vi "Configure Function FFT.vi"(6 "FFT Window (Hanning)":string(combo)="HANN", 8 "error in (no error)":errorcluster {"code" format="%.0x"}, 9 "fft center (500.0E+3 Hz)":dbl=500000.0 caption="FFT Center (500.0E+3 Hz)" format="%^.2e", 10 "fft span (1.0E+6 hz)":dbl=1000000.0 caption="FFT Span (1.0E+6 Hz)" format="%^.2e", 11 "VISA Resource Name":refnum<visa-resource-name>) -> (0 "error out":errorcluster {"code" format="%.0x"}, 3 "VISA Resource Name Out":refnum<visa-resource-name>)   [LabVIEW 2011, in "Agilent 546XX Series.lvlib"]
doc: "This VI configures the span, center and window values for the FFT function.\n\nNote: This VI has effects on the instrument only if the function operation is set to FFT."
uses:
  Agilent 546XX Series.lvlib
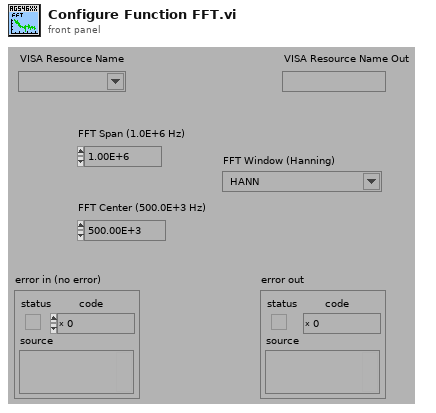
[diagram p1: front panel]
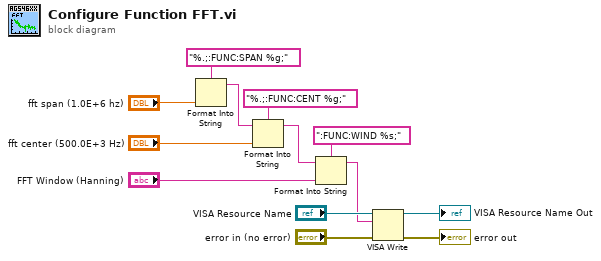
[diagram p0: block diagram]
diagram:
  n1 = Format Into String(format string="%.;:FUNC:SPAN %g;", "fft span (1.0E+6 hz)") -> (resulting string=w6:string)  [unwired: 2 in, 1 out]
  n2 = Format Into String(format string="%.;:FUNC:CENT %g;", initial string=w6, "fft center (500.0E+3 Hz)") -> (resulting string=w3:string)  [unwired: 1 in, 1 out]
  n3 = Format Into String(format string=":FUNC:WIND %s;", initial string=w3, "FFT Window (Hanning)") -> (resulting string=w1:string)  [unwired: 1 in, 1 out]
  n4 = VISA Write(VISA resource name="VISA Resource Name", write buffer=w1, error in (no error)="error in (no error)") -> (VISA resource name out=→"VISA Resource Name Out":refnum<visa-resource-name>, error out=→"error out":errorcluster)  [unwired: 1 out]
